vi "StageMoveDone.vi"(8 "error in (no error)":errorcluster, 10 "Positions":T1={"CH1 Pos"=0.0, "CH2 Pos"=0.0, "CH3 Pos"=0.0, "CH4 Pos"=0.0, "Home?"=TRUE}, 11 "Arduino_TranslationStage_UI.lvlib:Arduino_Stepper.lvclass":refnum<class "Arduino_Stepper_UI.lvclass">) -> (0 "error out":errorcluster, 3 "Arduino_TranslationStage_UI.lvlib:Arduino_Stepper.lvclass":refnum<class "Arduino_Stepper_UI.lvclass">)   [LabVIEW 2023, in "Arduino_TranslationStage_UI.lvlib" / "Arduino_Stepper_UI.lvclass"]
uses:
  Arduino_Stepper_UI.lvclass
  TranslationStage_UI/TranslationStage_UI/StageMoveDone_For_UI.ctl
  typedefs/typedefs.lvlib
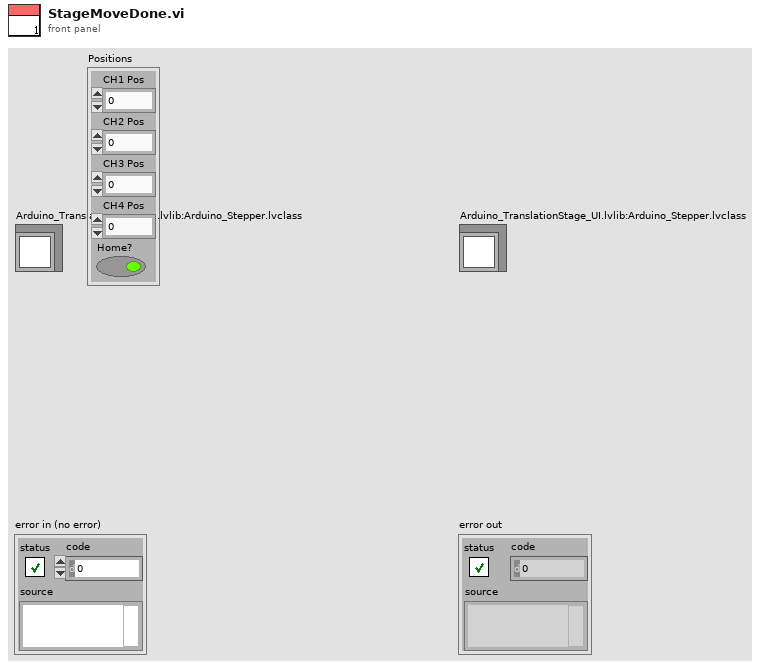
[diagram p1: front panel]
types:
  T1 = typedef "typedefs.lvlib/StageMoveDone_For_UI.ctl" = cluster{"CH1 Pos":sgl, "CH2 Pos":dbl, "CH3 Pos":dbl, "CH4 Pos":dbl, "Home?":bool}
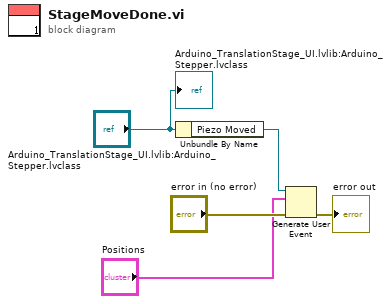
[diagram p0: block diagram]
diagram:
  n1 = Unbundle By Name("Arduino_TranslationStage_UI.lvlib:Arduino_Stepper.lvclass") -> ("Piezo Moved"=w4:refnum<user-event>)
  n2 = Generate User Event(user event=w4, event data cluster="Positions", error in="error in (no error)") -> (error out=→"error out":errorcluster)  [unwired: 1 in, 1 out]
  "Arduino_TranslationStage_UI.lvlib:Arduino_Stepper.lvclass" <- "Arduino_TranslationStage_UI.lvlib:Arduino_Stepper.lvclass"
